vi "HL_RR-4_In2O3.vi"() -> ()   [LabVIEW 2015]
uses:
  <vilib>/MakerHub/LINX/Public/Peripherals/Digital/Digital Write N Chans.vi
  <vilib>/MakerHub/LINX/Public/Peripherals/Analog/Analog Read 1 Chan.vi
  <vilib>/MakerHub/LINX/Private/Local IO/LinxDigitalWrite.vi
  <vilib>/MakerHub/LINX/Public/Utilities/Check Channel.vi
  <vilib>/MakerHub/LINX/Public/Peripherals/Analog/Analog Read N Chans.vi
  <vilib>/MakerHub/LINX/Private/Local IO/LinxAnalogRead.vi
  <vilib>/MakerHub/LINX/Public/Utilities/Open Serial.vi
  <vilib>/MakerHub/LINX/Private/Utilties/Generate Error.vi
  <vilib>/MakerHub/LINX/LMH-LINX.lvlib
panel:
  in  "high R - 2":dbl
  in  "time post":u32
  in  "number of pulses":i32
  in  "low R - 2":dbl
  out "Ref":dbl(graph)
  in  "LED":refnum<visa-resource-name>="N/A"
  out "3":dbl(graph)
  out "2":dbl(graph)
  out "4":dbl(graph)
  out "1":dbl(graph)
  out "pos":dbl
  in  "milliseconds to wait":u32
  in  "time pre":u32
  in  "Serial Port Analog":refnum<visa-resource-name>="N/A"
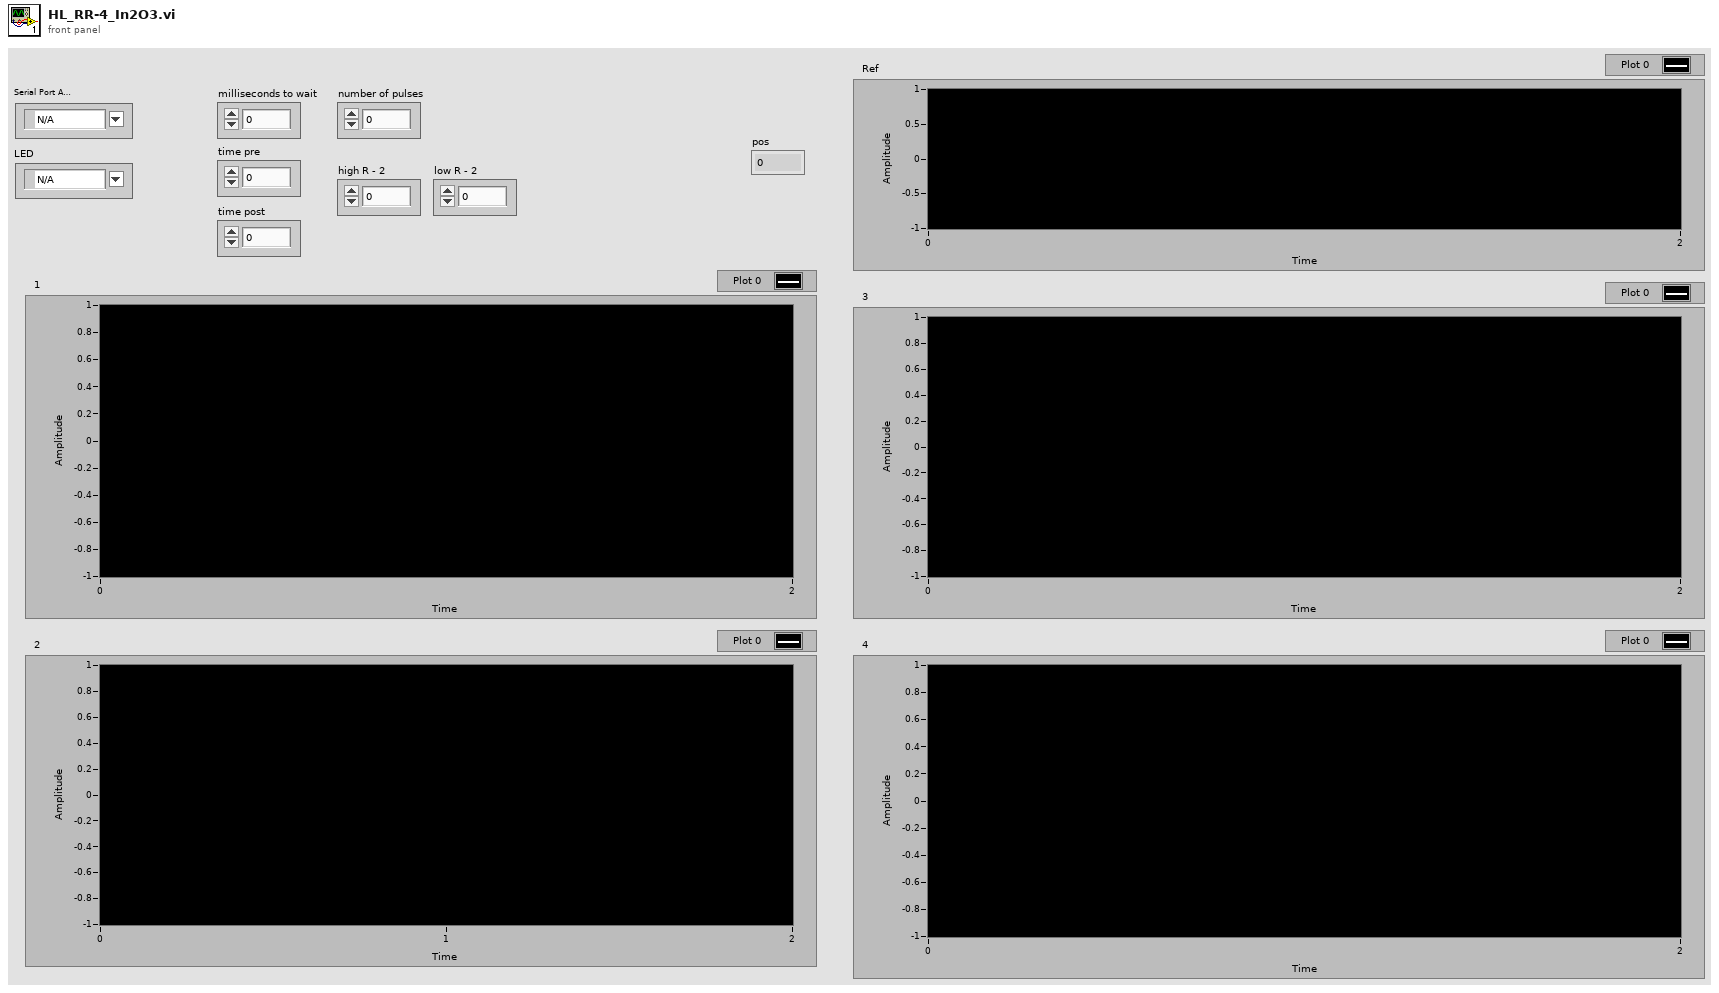
[diagram p1: front panel]
types:
  T1 = typedef "LMH-LINX.lvlib/LINX Ref.ctl" = cluster{"IO":T2, "Interface":T3, "LINX Device Config":T4}
  T2 = typedef "LMH-LINX.lvlib/Platform.ctl" = enum16{"Remote", "Local"}
  T3 = typedef "LMH-LINX.lvlib/Interface.ctl" = enum16{"Serial", "TCP"}
  T4 = typedef "LMH-LINX.lvlib/Device.lvlib/LINX Device Config.ctl" = cluster{"Interface":T3, "COM Port":refnum<visa-resource-name>, "TCP Configuration":T5, "Device Family":u8, "Device ID":u8, "Device Name":string, "TCP Ref":refnum<k5>, "Channels":T6}
  T5 = typedef "LMH-LINX.lvlib/Device.lvlib/TCP Config.ctl" = cluster{"IP Address":string, "Port":u16}
  T6 = typedef "LMH-LINX.lvlib/Channels.ctl" = cluster{"DI":u8[], "DO":u8[], "AI":u8[], "AO":u8[], "PWM":u8[], "QE":u8[], "UART":u8[], "I2C 2":u8[], "SPI":u8[], "CAN":u8[], "Servo":u8[], "AI Ref (V)":dbl, "AI Resolution (Bits)":u8, "AO Ref (V)":dbl, "AO Resolution (Bits)":u8}
  T7 = enum16{"open", "replace", "create", "open or create", "replace or create", "replace or create with confirmation"}
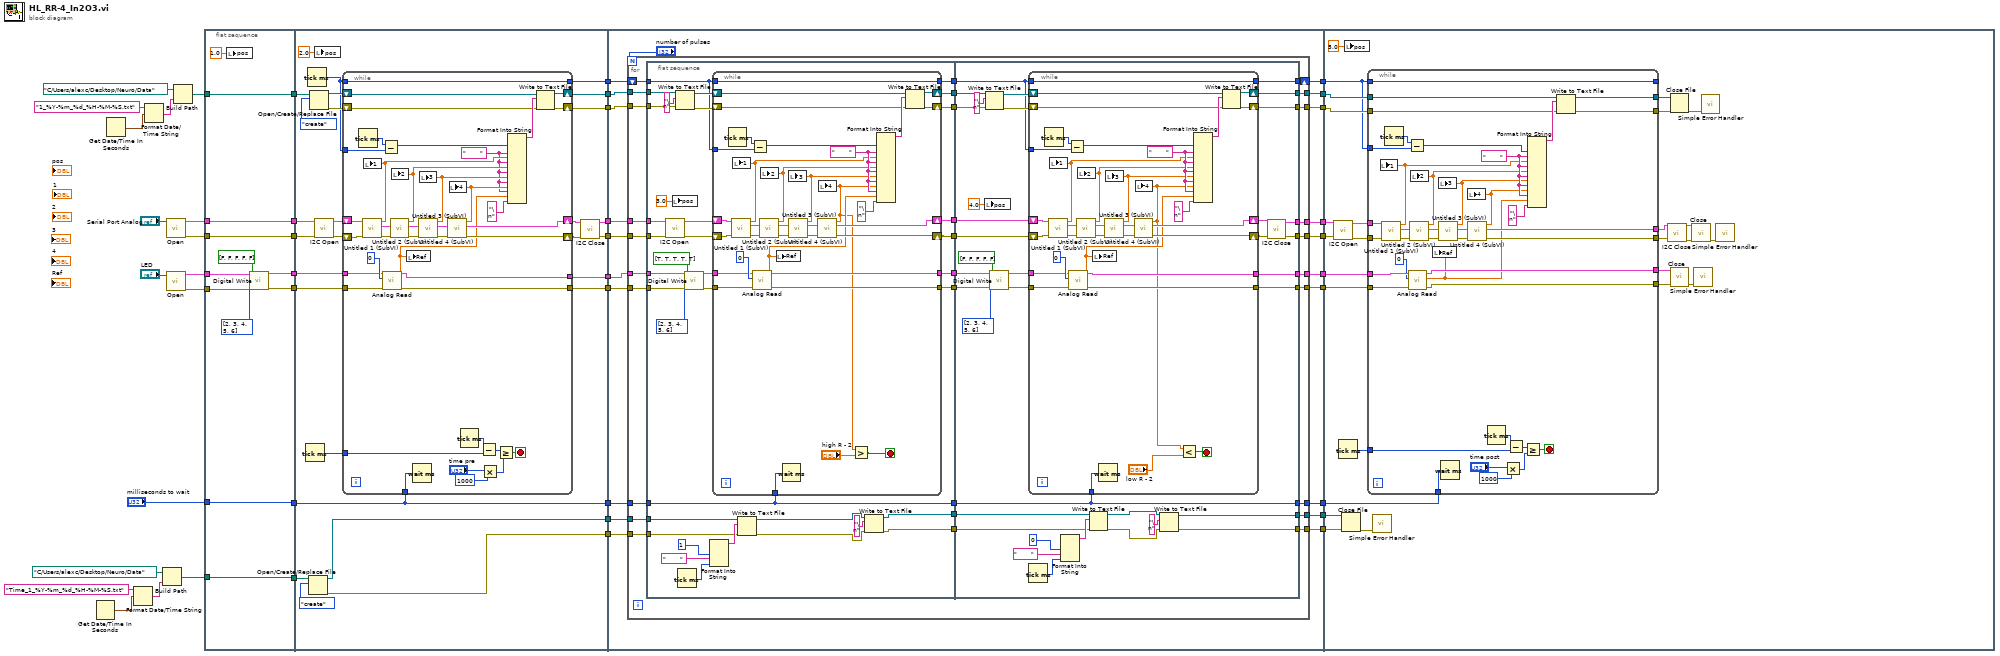
[diagram p0: block diagram]
diagram:
  n1 = Get Date/Time In Seconds() -> (seconds since 1Jan1904=w8:timestamp)
  n2 = Get Date/Time In Seconds() -> (seconds since 1Jan1904=w22:timestamp)
  n3 = Format Date/Time String(time format string (%c)="Time_1_%Y-%m_%d_%H-%M-%S.txt", seconds (now)=w8) -> (date/time string=w10:string)  [unwired: 1 in]
  n4 = Format Date/Time String(time format string (%c)="1_%Y-%m_%d_%H-%M-%S.txt", seconds (now)=w22) -> (date/time string=w24:string)  [unwired: 1 in]
  n5 = Build Path(base path=path "C:/Users/alexc/Desktop/Neuro/Data", name or relative path=w10) -> (appended path=w6:path)
  n6 = call-poly <vilib>:"Open.vi"("Serial Port"="Serial Port Analog") -> ("Error Out"=w28:errorcluster, "LINX Resource"=w29:T1)  [unwired: 8 in, 1 out]
  n7 = call-poly <vilib>:"Open.vi"("Serial Port"="LED") -> ("Error Out"=w19:errorcluster, "LINX Resource"=w20:T1)  [unwired: 8 in, 1 out]
  n8 = Build Path(base path=path "C:/Users/alexc/Desktop/Neuro/Data", name or relative path=w24) -> (appended path=w21:path)
  n9 = flat-sequence {
    tunnel: [w53] -> w44
    tunnel: [w52] -> w43
    tunnel: [w51] -> w40
    tunnel: [w46] -> w31
    tunnel: w29 -> [w53]
    tunnel: w28 -> [w52]
    tunnel: w21 -> [w51]
    tunnel: w20 -> [w50]
    tunnel: w19 -> [w49]
    tunnel: [w48] -> w18
    tunnel: [w47] -> w17
    tunnel: "milliseconds to wait" -> [w46]
    tunnel: [w45] -> w7
    tunnel: w6 -> [w45]
    tunnel: w44 -> [w83]
    tunnel: w43 -> [w82]
    tunnel: [w81] -> w42
    tunnel: [w80] -> w41
    tunnel: w40 -> [w79]
    tunnel: [w75] -> w39
    tunnel: [w74] -> w38
    tunnel: [w72] -> w37
    tunnel: w31 -> [w70]
    tunnel: [w70] -> w30
    tunnel: w18 -> [w64]
    tunnel: w17 -> [w63]
    tunnel: [w62] -> w16
    tunnel: w7 -> [w60]
    tunnel: [w59] -> w5
    tunnel: [w58] -> w4
    tunnel: [w57] -> w1
    tunnel: [w132] -> w36
    tunnel: [w131] -> w35
    tunnel: [w135] -> w34
    tunnel: [w134] -> w33
    tunnel: [w133] -> w32
    tunnel: w30 -> [w136]
    tunnel: w37 -> [w140]
    tunnel: w38 -> [w141]
    tunnel: w39 -> [w142]
    tunnel: w41 -> [w138]
    tunnel: w42 -> [w139]
    tunnel: w16 -> [w143]
    tunnel: [w130] -> w14
    tunnel: [w129] -> w13
    tunnel: [w128] -> w12
    tunnel: w5 -> [w127]
    tunnel: w4 -> [w126]
    tunnel: [w125] -> w3
    tunnel: [w124] -> w2
    tunnel: w1 -> [w123]
    tunnel: w32 -> [w330]
    tunnel: w33 -> [w331]
    tunnel: w34 -> [w317]
    tunnel: w35 -> [w335]
    tunnel: w36 -> [w339]
    tunnel: w14 -> [w334]
    tunnel: w13 -> [w321]
    tunnel: w12 -> [w320]
    tunnel: w3 -> [w315]
    tunnel: w2 -> [w314]
    frame #0 {
      n10 = local write "pos"(1.0 ("pos")) -> ()
      n11 = call-poly <vilib>:"Digital Write.vi"("Error In"=w49, "Values"=bool[] [FALSE, FALSE, FALSE, FALSE, FALSE], "DO Channels"=u8[] [2, 3, 4, 5, 6], "LINX Resource"=w50) -> ("Error Out"=w47:errorcluster, "LINX Resource"=w48:T1)  [unwired: 6 in]
    }
    frame #1 {
      n12 = Tick Count (ms)() -> (millisecond timer value=w71:u32)
      n13 = Tick Count (ms)() -> (millisecond timer value=w73:u32)
      n14 = Open/Create/Replace File(file path (use dialog)=w60, operation (0:open)=T7."create") -> (refnum out=w59:refnum<file>, error out=w58:errorcluster)  [unwired: 4 in, 1 out]
      n15 = Open/Create/Replace File(file path (use dialog)=w79, operation (0:open)=T7."create") -> (refnum out=w77:refnum<file>, error out=w76:errorcluster)  [unwired: 4 in, 1 out]
      n16 = local write "pos"(2.0 ("pos")) -> ()
      n17 = call <vilib>:"I2C Open.vi"("Error In"=w82, "LINX Resource"=w83) -> ("Error Out"=w68:errorcluster, "LINX Resource"=w69:T1)  [unwired: 8 in]
      n18 = while {
        tunnel: w73 -> [w115]
        shift-right: [w111] -> w75
        shift-left: w77 -> [w113]
        shift-right: [w110] -> w74
        shift-left: w76 -> [w112]
        tunnel: [w109] -> w72
        tunnel: w73 -> [w109]
        tunnel: w71 -> [w89]
        tunnel: w70 -> [w93]
        shift-right: [w106] -> w67
        shift-left: w69 -> [w108]
        shift-right: [w105] -> w66
        shift-left: w68 -> [w107]
        tunnel: w64 -> [w95]
        tunnel: w63 -> [w94]
        tunnel: [w92] -> w62
        tunnel: [w84] -> w57
        stop <- w88 stop-if-true
        w99 = "       "
        n19 = Tick Count (ms)() -> (millisecond timer value=w116:u32)
        n20 = call "Untitled 1 (SubVI).vi"("error in (no error)"=w107, "LINX Resource in"=w108) -> ("error out"=w121:errorcluster, "LINX Resource out"=w122:T1, "Numeric"=w103:dbl)  [unwired: 7 in]
        n21 = local write "1"(w103) -> ()
        n22 = Subtract(x=w116, y=w115) -> (x-y=w100:u32)
        n23 = call-poly <vilib>:"Analog Read.vi"("Error In"=w94, "Analog Channel"=u8 0, "LINX Resource"=w95) -> ("Error Out"=w84:errorcluster, "Voltage"=w96:dbl, "LINX Resource"=w92:T1)  [unwired: 5 in, 1 out]
        n24 = call "Untitled 2 (SubVI).vi"("error in (no error)"=w121, "LINX Resource in"=w122) -> ("error out"=w120:errorcluster, "LINX Resource"=w119:T1, "Numeric"=w102:dbl)  [unwired: 7 in]
        n25 = local write "2"(w102) -> ()
        n26 = local write "Ref"(w96) -> ()
        n27 = Wait (ms)(milliseconds to wait=w93) -> ()  [unwired: 1 out]
        n28 = call "Untitled 3 (SubVI).vi"("error in (no error)"=w120, "LINX Resource in"=w119) -> ("error out"=w117:errorcluster, "LINX Resource out"=w118:T1, "Numeric"=w101:dbl)  [unwired: 7 in]
        n29 = local write "3"(w101) -> ()
        n30 = call "Untitled 4 (SubVI).vi"("error in (no error)"=w117, "LINX Resource in"=w118) -> ("error out"=w105:errorcluster, "LINX Resource"=w106:T1, "Numeric"=w104:dbl)  [unwired: 7 in]
        n31 = local write "4"(w104) -> ()
        n32 = Tick Count (ms)() -> (millisecond timer value=w90:u32)
        n33 = Subtract(x=w90, y=w89) -> (x-y=w91:u32)
        n34 = Multiply(x="time pre", y=u32 1000) -> (x*y=w87:u32)
        n35 = Greater Or Equal?(x=w91, y=w87) -> (x >= y?=w88:bool)
        n36 = Format Into String(w100, w99, w103, w99, w102, w99, w101, w99, w104, w99, w96, "\n") -> (resulting string=w114:string)  [unwired: 3 in, 1 out]
        n37 = Write to Text File(file (use dialog)=w113, text=w114, error in=w112) -> (refnum out=w111:refnum<file>, error out=w110:errorcluster)  [unwired: 1 in, 1 out]
      }
      n38 = call <vilib>:"I2C Close.vi"("Error In"=w66, "LINX Resource"=w67) -> ("Error Out"=w80:errorcluster, "LINX Resource"=w81:T1)  [unwired: 8 in]
    }
    frame #2 {
      n39 = for {
        N: "number of pulses" -> [_]
        tunnel: w143 -> [w173]
        tunnel: w142 -> [w172]
        tunnel: w141 -> [w171]
        shift-right: [w158] -> w135
        shift-left: w140 -> [w168]
        tunnel: w139 -> [w170]
        tunnel: w138 -> [w169]
        tunnel: w136 -> [w160]
        tunnel: [w157] -> w134
        tunnel: [w156] -> w133
        tunnel: [w155] -> w132
        tunnel: [w154] -> w131
        tunnel: [w153] -> w130
        tunnel: [w152] -> w129
        tunnel: [w151] -> w128
        tunnel: w127 -> [w150]
        tunnel: w126 -> [w149]
        tunnel: [w146] -> w125
        tunnel: [w145] -> w124
        tunnel: w123 -> [w144]
        n40 = flat-sequence {
          tunnel: w173 -> [w204]
          tunnel: w172 -> [w201]
          tunnel: w171 -> [w200]
          tunnel: w170 -> [w193]
          tunnel: w169 -> [w192]
          tunnel: w168 -> [w189]
          tunnel: [w208] -> w167
          tunnel: [w207] -> w166
          tunnel: [w203] -> w165
          tunnel: [w202] -> w164
          tunnel: [w197] -> w163
          tunnel: [w196] -> w162
          tunnel: [w188] -> w161
          tunnel: w160 -> [w186]
          tunnel: [w186] -> w159
          tunnel: w150 -> [w184]
          tunnel: w149 -> [w183]
          tunnel: [w176] -> w148
          tunnel: [w175] -> w147
          tunnel: w144 -> [w174]
          tunnel: w167 -> [w272]
          tunnel: w166 -> [w271]
          tunnel: w165 -> [w266]
          tunnel: w164 -> [w265]
          tunnel: w163 -> [w268]
          tunnel: w162 -> [w267]
          tunnel: w161 -> [w264]
          tunnel: w159 -> [w257]
          tunnel: [w262] -> w158
          tunnel: [w261] -> w157
          tunnel: [w260] -> w156
          tunnel: [w259] -> w155
          tunnel: [w258] -> w154
          tunnel: [w257] -> w153
          tunnel: [w256] -> w152
          tunnel: [w255] -> w151
          tunnel: w148 -> [w250]
          tunnel: w147 -> [w249]
          tunnel: [w245] -> w146
          tunnel: [w244] -> w145
          frame #0 {
            n41 = call <vilib>:"I2C Open.vi"("Error In"=w192, "LINX Resource"=w193) -> ("Error Out"=w190:errorcluster, "LINX Resource"=w191:T1)  [unwired: 8 in]
            n42 = local write "pos"(3.0 ("pos")) -> ()
            n43 = Write to Text File(file (use dialog)=w201, text="\n", error in=w200) -> (refnum out=w199:refnum<file>, error out=w198:errorcluster)  [unwired: 1 in, 1 out]
            n44 = Tick Count (ms)() -> (millisecond timer value=w180:u32)
            n45 = call-poly <vilib>:"Digital Write.vi"("Error In"=w174, "Values"=bool[] [TRUE, TRUE, TRUE, TRUE, TRUE], "DO Channels"=u8[] [2, 3, 4, 5, 6], "LINX Resource"=w204) -> ("Error Out"=w195:errorcluster, "LINX Resource"=w194:T1)  [unwired: 6 in]
            n46 = Format Into String(u32 1 ("input 1"), "       ", w180) -> (resulting string=w185:string)  [unwired: 3 in, 1 out]
            n47 = while {
              tunnel: w189 -> [w236]
              shift-right: [w232] -> w203
              shift-left: w199 -> [w234]
              shift-right: [w231] -> w202
              shift-left: w198 -> [w233]
              tunnel: [w230] -> w188
              tunnel: w189 -> [w230]
              tunnel: w186 -> [w218]
              shift-right: [w227] -> w208
              shift-left: w191 -> [w229]
              shift-right: [w226] -> w207
              shift-left: w190 -> [w228]
              tunnel: w194 -> [w220]
              tunnel: w195 -> [w219]
              tunnel: [w217] -> w197
              tunnel: [w216] -> w196
              stop <- w215 stop-if-true
              w224 = "       "
              n48 = Tick Count (ms)() -> (millisecond timer value=w237:u32)
              n49 = call "Untitled 1 (SubVI).vi"("error in (no error)"=w228, "LINX Resource in"=w229) -> ("error out"=w242:errorcluster, "LINX Resource out"=w243:T1, "Numeric"=w214:dbl)  [unwired: 7 in]
              n50 = local write "1"(w214) -> ()
              n51 = Subtract(x=w237, y=w236) -> (x-y=w225:u32)
              n52 = call-poly <vilib>:"Analog Read.vi"("Error In"=w219, "Analog Channel"=u8 0, "LINX Resource"=w220) -> ("Error Out"=w216:errorcluster, "Voltage"=w221:dbl, "LINX Resource"=w217:T1)  [unwired: 5 in, 1 out]
              n53 = call "Untitled 2 (SubVI).vi"("error in (no error)"=w242, "LINX Resource in"=w243) -> ("error out"=w241:errorcluster, "LINX Resource"=w240:T1, "Numeric"=w212:dbl)  [unwired: 7 in]
              n54 = local write "2"(w212) -> ()
              n55 = local write "Ref"(w221) -> ()
              n56 = Wait (ms)(milliseconds to wait=w218) -> ()  [unwired: 1 out]
              n57 = call "Untitled 3 (SubVI).vi"("error in (no error)"=w241, "LINX Resource in"=w240) -> ("error out"=w238:errorcluster, "LINX Resource out"=w239:T1, "Numeric"=w211:dbl)  [unwired: 7 in]
              n58 = local write "3"(w211) -> ()
              n59 = call "Untitled 4 (SubVI).vi"("error in (no error)"=w238, "LINX Resource in"=w239) -> ("error out"=w226:errorcluster, "LINX Resource"=w227:T1, "Numeric"=w210:dbl)  [unwired: 7 in]
              n60 = local write "4"(w210) -> ()
              n61 = Greater?(x=w210, y="high R - 2") -> (0:w215:bool)
              n62 = Format Into String(w225, w224, w214, w224, w212, w224, w211, w224, w210, w224, w221, "\n") -> (resulting string=w235:string)  [unwired: 3 in, 1 out]
              n63 = Write to Text File(file (use dialog)=w234, text=w235, error in=w233) -> (refnum out=w232:refnum<file>, error out=w231:errorcluster)  [unwired: 1 in, 1 out]
            }
            n64 = Write to Text File(file (use dialog)=w184, text=w185, error in=w183) -> (refnum out=w178:refnum<file>, error out=w177:errorcluster)  [unwired: 1 in, 1 out]
            n65 = Write to Text File(file (use dialog)=w178, text="\n", error in=w177) -> (refnum out=w176:refnum<file>, error out=w175:errorcluster)  [unwired: 1 in, 1 out]
          }
          frame #1 {
            n66 = local write "pos"(4.0 ("pos")) -> ()
            n67 = Write to Text File(file (use dialog)=w266, text="\n", error in=w265) -> (refnum out=w274:refnum<file>, error out=w275:errorcluster)  [unwired: 1 in, 1 out]
            n68 = call-poly <vilib>:"Digital Write.vi"("Error In"=w267, "Values"=bool[] [FALSE, FALSE, FALSE, FALSE, FALSE], "DO Channels"=u8[] [2, 3, 4, 5, 6], "LINX Resource"=w268) -> ("Error Out"=w279:errorcluster, "LINX Resource"=w278:T1)  [unwired: 6 in]
            n69 = while {
              tunnel: w264 -> [w306]
              shift-right: [w302] -> w261
              shift-left: w274 -> [w304]
              shift-right: [w301] -> w260
              shift-left: w275 -> [w303]
              tunnel: [w300] -> w262
              tunnel: w264 -> [w300]
              tunnel: w257 -> [w288]
              shift-right: [w297] -> w270
              shift-left: w272 -> [w299]
              shift-right: [w296] -> w269
              shift-left: w271 -> [w298]
              tunnel: w278 -> [w290]
              tunnel: w279 -> [w289]
              tunnel: [w287] -> w256
              tunnel: [w286] -> w255
              stop <- w285 stop-if-true
              w294 = "       "
              n70 = Tick Count (ms)() -> (millisecond timer value=w307:u32)
              n71 = call "Untitled 1 (SubVI).vi"("error in (no error)"=w298, "LINX Resource in"=w299) -> ("error out"=w312:errorcluster, "LINX Resource out"=w313:T1, "Numeric"=w283:dbl)  [unwired: 7 in]
              n72 = local write "1"(w283) -> ()
              n73 = Subtract(x=w307, y=w306) -> (x-y=w295:u32)
              n74 = call-poly <vilib>:"Analog Read.vi"("Error In"=w289, "Analog Channel"=u8 0, "LINX Resource"=w290) -> ("Error Out"=w286:errorcluster, "Voltage"=w291:dbl, "LINX Resource"=w287:T1)  [unwired: 5 in, 1 out]
              n75 = call "Untitled 2 (SubVI).vi"("error in (no error)"=w312, "LINX Resource in"=w313) -> ("error out"=w311:errorcluster, "LINX Resource"=w310:T1, "Numeric"=w282:dbl)  [unwired: 7 in]
              n76 = local write "2"(w282) -> ()
              n77 = local write "Ref"(w291) -> ()
              n78 = Wait (ms)(milliseconds to wait=w288) -> ()  [unwired: 1 out]
              n79 = call "Untitled 3 (SubVI).vi"("error in (no error)"=w311, "LINX Resource in"=w310) -> ("error out"=w308:errorcluster, "LINX Resource out"=w309:T1, "Numeric"=w281:dbl)  [unwired: 7 in]
              n80 = local write "3"(w281) -> ()
              n81 = call "Untitled 4 (SubVI).vi"("error in (no error)"=w308, "LINX Resource in"=w309) -> ("error out"=w296:errorcluster, "LINX Resource"=w297:T1, "Numeric"=w280:dbl)  [unwired: 7 in]
              n82 = local write "4"(w280) -> ()
              n83 = Less?(x=w280, y="low R - 2") -> (x < y?=w285:bool)
              n84 = Format Into String(w295, w294, w283, w294, w282, w294, w281, w294, w280, w294, w291, "\n") -> (resulting string=w305:string)  [unwired: 3 in, 1 out]
              n85 = Write to Text File(file (use dialog)=w304, text=w305, error in=w303) -> (refnum out=w302:refnum<file>, error out=w301:errorcluster)  [unwired: 1 in, 1 out]
            }
            n86 = Tick Count (ms)() -> (millisecond timer value=w251:u32)
            n87 = Format Into String(u32 0 ("input 1"), "       ", w251) -> (resulting string=w254:string)  [unwired: 3 in, 1 out]
            n88 = Write to Text File(file (use dialog)=w250, text=w254, error in=w249) -> (refnum out=w247:refnum<file>, error out=w246:errorcluster)  [unwired: 1 in, 1 out]
            n89 = Write to Text File(file (use dialog)=w247, text="\n", error in=w246) -> (refnum out=w245:refnum<file>, error out=w244:errorcluster)  [unwired: 1 in, 1 out]
            n90 = call <vilib>:"I2C Close.vi"("Error In"=w269, "LINX Resource"=w270) -> ("Error Out"=w258:errorcluster, "LINX Resource"=w259:T1)  [unwired: 8 in]
          }
        }
      }
    }
    frame #3 {
      n91 = call <vilib>:"I2C Open.vi"("Error In"=w335, "LINX Resource"=w339) -> ("Error Out"=w332:errorcluster, "LINX Resource"=w333:T1)  [unwired: 8 in]
      n92 = Tick Count (ms)() -> (millisecond timer value=w329:u32)
      n93 = Close File(refnum=w315, error in=w314) -> (error out=w316:errorcluster)  [unwired: 1 out]
      n94 = local write "pos"(5.0 ("pos")) -> ()
      n95 = while {
        tunnel: w334 -> [w372]
        tunnel: w333 -> [w371]
        tunnel: w332 -> [w370]
        tunnel: [w364] -> _
        tunnel: w317 -> [w364]
        tunnel: w331 -> [w363]
        tunnel: w330 -> [w362]
        tunnel: w329 -> [w343]
        tunnel: [w361] -> w328
        tunnel: [w360] -> w327
        tunnel: [w359] -> w324
        tunnel: [w358] -> w323
        tunnel: w321 -> [w357]
        tunnel: w320 -> [w356]
        tunnel: [w355] -> w319
        tunnel: [w354] -> w318
        tunnel: w317 -> [w352]
        stop <- w344 stop-if-true
        w374 = "       "
        n96 = call "Untitled 1 (SubVI).vi"("error in (no error)"=w370, "LINX Resource in"=w371) -> ("error out"=w369:errorcluster, "LINX Resource out"=w378:T1, "Numeric"=w366:dbl)  [unwired: 7 in]
        n97 = local write "1"(w366) -> ()
        n98 = Tick Count (ms)() -> (millisecond timer value=w365:u32)
        n99 = Subtract(x=w365, y=w352) -> (x-y=w351:u32)
        n100 = call-poly <vilib>:"Analog Read.vi"("Error In"=w356, "Analog Channel"=u8 0, "LINX Resource"=w357) -> ("Error Out"=w354:errorcluster, "Voltage"=w350:dbl, "LINX Resource"=w355:T1)  [unwired: 5 in, 1 out]
        n101 = call "Untitled 2 (SubVI).vi"("error in (no error)"=w369, "LINX Resource in"=w378) -> ("error out"=w368:errorcluster, "LINX Resource"=w377:T1, "Numeric"=w349:dbl)  [unwired: 7 in]
        n102 = local write "2"(w349) -> ()
        n103 = local write "Ref"(w350) -> ()
        n104 = call "Untitled 3 (SubVI).vi"("error in (no error)"=w368, "LINX Resource in"=w377) -> ("error out"=w367:errorcluster, "LINX Resource out"=w376:T1, "Numeric"=w348:dbl)  [unwired: 7 in]
        n105 = local write "3"(w348) -> ()
        n106 = Wait (ms)(milliseconds to wait=w372) -> ()  [unwired: 1 out]
        n107 = call "Untitled 4 (SubVI).vi"("error in (no error)"=w367, "LINX Resource in"=w376) -> ("error out"=w358:errorcluster, "LINX Resource"=w359:T1, "Numeric"=w347:dbl)  [unwired: 7 in]
        n108 = local write "4"(w347) -> ()
        n109 = Tick Count (ms)() -> (millisecond timer value=w345:u32)
        n110 = Multiply(x="time post", y=u32 1000) -> (x*y=w342:u32)
        n111 = Subtract(x=w345, y=w343) -> (x-y=w346:u32)
        n112 = Greater Or Equal?(x=w346, y=w342) -> (x >= y?=w344:bool)
        n113 = Format Into String(w351, w374, w366, w374, w349, w374, w348, w374, w347, w374, w350, "\n") -> (resulting string=w375:string)  [unwired: 3 in, 1 out]
        n114 = Write to Text File(file (use dialog)=w363, text=w375, error in=w362) -> (refnum out=w361:refnum<file>, error out=w360:errorcluster)  [unwired: 1 in, 1 out]
      }
      n115 = call <vilib>:"Simple Error Handler.vi"("error in (no error)"=w316) -> ()  [unwired: 4 in, 5 out]
      n116 = call <vilib>:"I2C Close.vi"("Error In"=w323, "LINX Resource"=w324) -> ("Error Out"=w325:errorcluster, "LINX Resource"=w326:T1)  [unwired: 8 in]
      n117 = Close File(refnum=w328, error in=w327) -> (error out=w338:errorcluster)  [unwired: 1 out]
      n118 = call <vilib>:"Close.vi"("Error In"=w318, "LINX Resource"=w319) -> ("Error Out"=w322:errorcluster)  [unwired: 9 in]
      n119 = call <vilib>:"Close.vi"("Error In"=w325, "LINX Resource"=w326) -> ("Error Out"=w337:errorcluster)  [unwired: 9 in]
      n120 = call <vilib>:"Simple Error Handler.vi"("error in (no error)"=w322) -> ()  [unwired: 4 in, 5 out]
      n121 = call <vilib>:"Simple Error Handler.vi"("error in (no error)"=w338) -> ()  [unwired: 4 in, 5 out]
      n122 = call <vilib>:"Simple Error Handler.vi"("error in (no error)"=w337) -> ()  [unwired: 4 in, 5 out]
    }
  }
